vi "1 - Event API Syntax and Semantics.vi"   [LabVIEW 2012]
panel:
  # "User Events Tips, Tricks, and Sundry"
  # "Jack Dunaway - CLA - LabVIEW Champion"
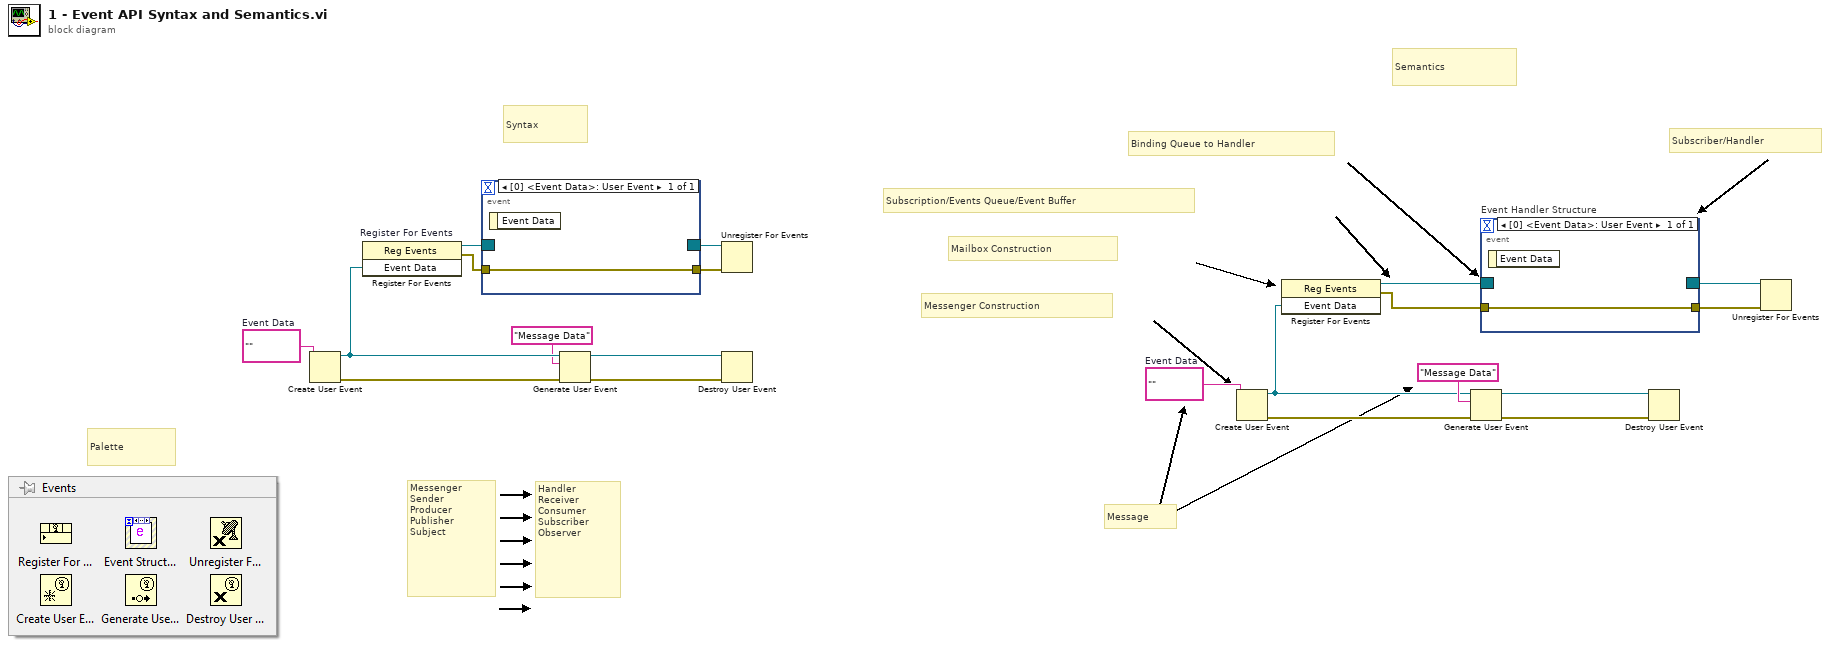
[diagram p0: block diagram]
diagram:
  w6 = ""  # Event Data
  w15 = ""  # Event Data
  # "Messenger Construction"
  # "Binding Queue to Handler"
  # "Handler\nReceiver\nConsumer\nSubscriber\nObserver"
  # "Messenger\nSender\nProducer\nPublisher\nSubject"
  # "Subscriber/Handler"
  # "Mailbox Construction"
  # "Message"
  # "Subscription/Events Queue/Event Buffer"
  # "Semantics"
  # "Palette"
  # "Syntax"
  n1 = Create User Event(user event datatype=w15) -> (user event=w19:refnum<user-event>, error out=w16:errorcluster)  [unwired: 1 in]
  n2 = register-events "Register For Events"(w19) -> (reference out=w20:refnum<event-registration>, error out=w13:errorcluster)  [unwired: 2 in]
  n3 = event shown="[0] <Event Data>: User Event" {
    selector: w20 -> [_]
    dyn-events: [_] -> w14
    timeout: _ -> [_]
    tunnel: w13 -> [w21]
    tunnel: [w21] -> w12
    event User Event {
      n4 = event-data() -> ()  [unwired: 1 in, 1 out]
    }
  }
  n5 = Generate User Event(user event=w19, event data cluster="Message Data" ("event data"), error in=w16) -> (user event out=w18:refnum<user-event>, error out=w17:errorcluster)
  n6 = Unregister For Events(event registration refnum=w14, error in=w12) -> ()  [unwired: 1 out]
  n7 = Destroy User Event(user event=w18, error in=w17) -> ()  [unwired: 1 out]
  n8 = Create User Event(user event datatype=w6) -> (user event=w2:refnum<user-event>, error out=w5:errorcluster)  [unwired: 1 in]
  n9 = register-events(w2) -> (reference out=w1:refnum<event-registration>, error out=w8:errorcluster)  [unwired: 2 in]
  n10 = Generate User Event(user event=w2, event data cluster="Message Data" ("event data"), error in=w5) -> (user event out=w3:refnum<user-event>, error out=w4:errorcluster)
  n11 = event "Event Handler Structure" shown="[0] <Event Data>: User Event" {
    selector: w1 -> [_]
    dyn-events: [_] -> w7
    timeout: _ -> [_]
    tunnel: w8 -> [w22]
    tunnel: [w22] -> w9
    event User Event {
      n12 = event-data() -> ()  [unwired: 1 in, 1 out]
    }
  }
  n13 = Destroy User Event(user event=w3, error in=w4) -> ()  [unwired: 1 out]
  n14 = Unregister For Events(event registration refnum=w7, error in=w9) -> ()  [unwired: 1 out]
